vi "Main.vi"() -> ()   [LabVIEW 2023]
panel:
  in  "User interface":T1(tab)
  in  "User entries":enum32{""}(tab)
  in  "Customization":enum32{"Customization"}(tab)
  in  "Marker shape":string
  in  "Marker size":i32
  in  "Open PDF":bool=TRUE
  in  "Open in MATLAB":bool=TRUE
  in  "Colors":enum32{"Colors"}(tab)
  out "Corners":u32(colorbox)
  out "Traces":u32[](array[colorbox])
  in  "Size":enum32{"Size"}(tab)
  out "Depth":i32
  out "Width":i16
  out "Height":i16
  out "stdout":string
  in  "PNG file path":path
  out "PNG picture":picture
  out "Traces.txt":string
  out "Script.m":string
  in  "Arrays":enum32{"Arrays"}(tab)
  out "Pixels colors (uchar)":u32[](array[numeric])
  out "Pixels colors (CLUT)":u8[](array[numeric])
  out "Corners color (CLUT)":i32
  out "Traces colors (RGB)":u8[][](array[numeric])
  out "Traces colors (CLUT)":i32[](array[numeric])
  out "Traces colors string (RGB)":string[](array[string])
  out "Number of Traces":i32
  out "Current VI folder":path
  out "PNG file name":string
  out "Pixmap.bin path":path
  out "Traces.txt path":path
  out "Extract path":path
  out "Script.m path":path
  out "PDF file path":path
  in  "MATLAB":enum32{"CallMATALB"}(tab)
  out "CallMATLAB out":errorcluster
  in  "C 2":enum32{"PNGFile"}(tab)
  out "PNGFile error":errorcluster
  in  "C 3":enum32{"PixmapWrite"}(tab)
  out "PixmapWrite error":errorcluster
  in  "C":enum32{"CallExtract"}(tab)
  out "CallExtract error 2":errorcluster
  out "CallExtract error":errorcluster
  in  "C 4":enum32{"TracesRead"}(tab)
  out "TracesRead error":errorcluster
  in  "C 5":enum32{"ScriptWrite"}(tab)
  out "ScriptWrite error":errorcluster
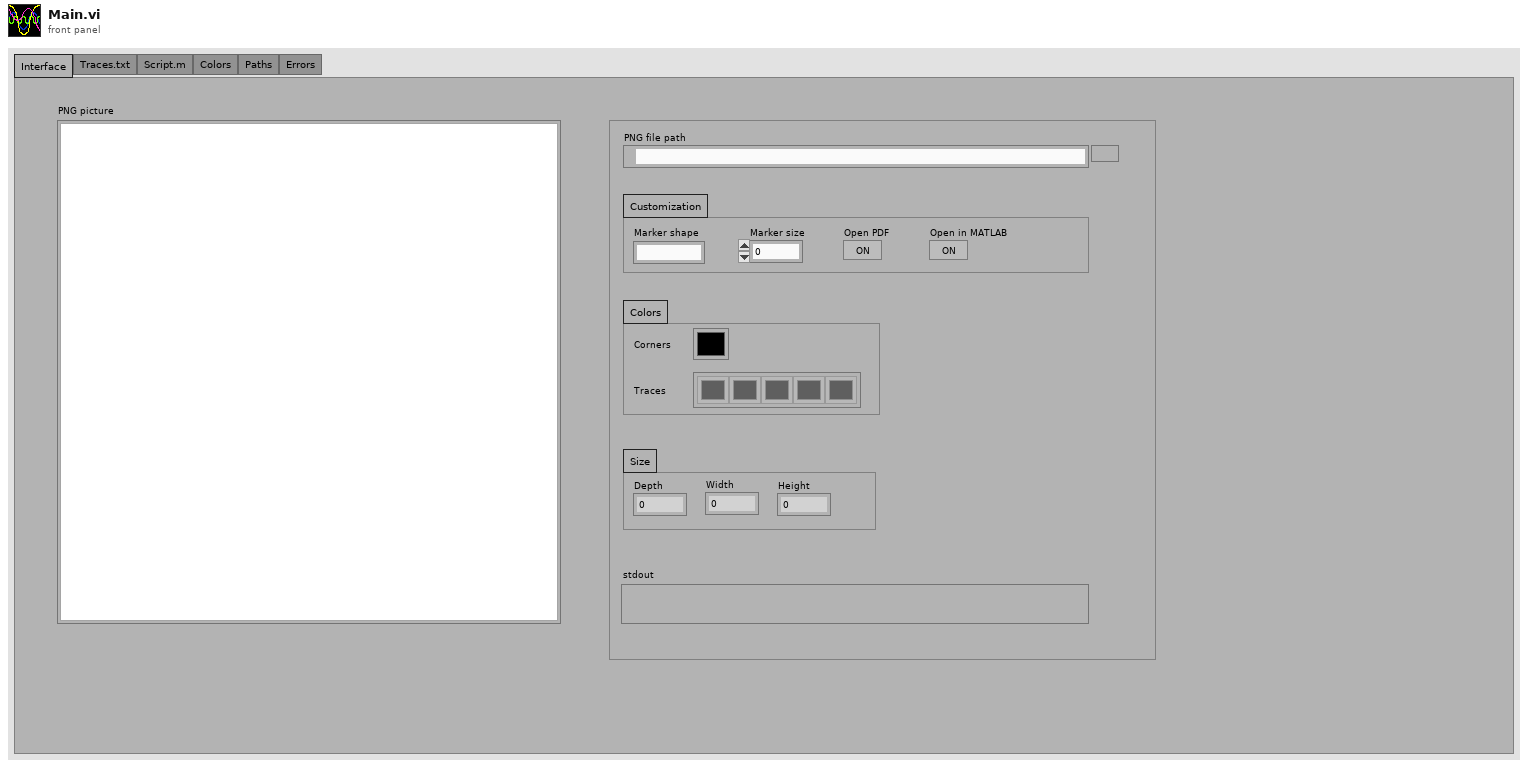
[diagram p1: front panel]
types:
  T1 = enum32{"Interface", "Traces.txt", "Script.m", "Colors", "Paths", "Errors"}
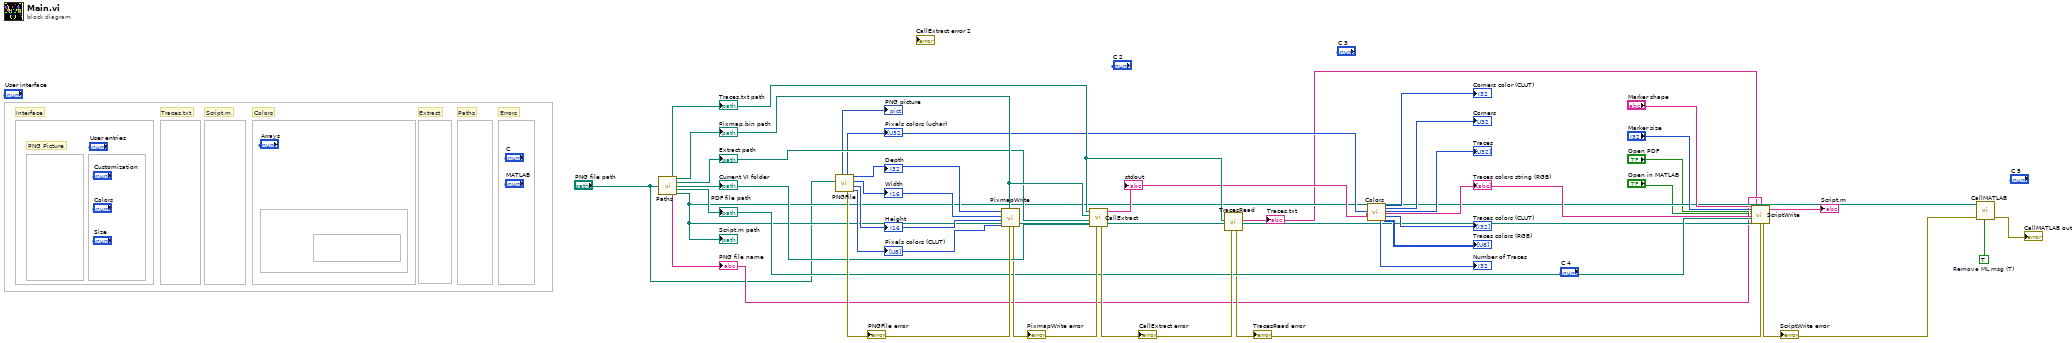
[diagram p0: block diagram]
diagram:
  w34 = TRUE  # Remove ML msg (T)
  # "PNG Picture"
  # "Errors"
  # "Paths"
  # "Extract"
  # "Colors"
  # "Script.m"
  # "Traces.txt"
  # "Interface"
  n1 = call "Paths.vi"("PNG file path"="PNG file path") -> ("Traces.txt path"=w24:path, "Pixmap.bin path"=w28:path, "Extract path"=w27:path, "VI folder"=w26:path, "PDF file path"=w10:path, "PNG file name"=w7:string, "Script.m path"=w9:path)  [unwired: 8 in]
  "Traces.txt path" <- w24
  "Pixmap.bin path" <- w28
  "Extract path" <- w27
  "Current VI folder" <- w26
  "PDF file path" <- w10
  "Script.m path" <- w9
  "PNG file name" <- w7
  n2 = call "PNGFile.vi"("PNG file path"="PNG file path") -> ("Pixels colors (CLUT)"=w30:u8[], "Height"=w31:i16, "Width"=w32:i16, "Depth"=w33:i32, "PNGFile error"=w29:errorcluster, "Pixels colors (uchar)"=w22:u32[], "PNG picture"=→"PNG picture":picture)  [unwired: 4 in]
  "Pixels colors (uchar)" <- w22
  "Depth" <- w33
  "Width" <- w32
  "Height" <- w31
  "Pixels colors (CLUT)" <- w30
  "PNGFile error" <- w29
  n3 = call "PixmapWrite.vi"("PNGFile error in"=w29, "Pixmap.bin path"=w28, "Pixels colors (CLUT)"=w30, "Height"=w31, "Width"=w32, "Depth"=w33) -> ("Pixmap.bin error out"=w25:errorcluster)  [unwired: 5 in]
  "PixmapWrite error" <- w25
  n4 = call "CallExtract.vi"("TracesWrite error"=w25, "VI folder"=w26, "Extract path"=w27, "Pixmap.bin path"=w28, "Traces.txt path"=w24) -> ("stdout"=w21:string, "CallExtract error"=w23:errorcluster)  [unwired: 4 in, 1 out]
  "CallExtract error" <- w23
  "stdout" <- w21
  n5 = call "TracesRead.vi"("Extract error"=w23, "Traces.txt path"=w24) -> ("Traces.txt"=w6:string, "TracesRead error"=w8:errorcluster)  [unwired: 8 in]
  "TracesRead error" <- w8
  "Traces.txt" <- w6
  n6 = call "Colors.vi"("Pixels colors (uchar)"=w22, "stdout"=w21) -> ("Number of Traces"=→"Number of Traces":i32, "Corners color (CLUT)"=→"Corners color (CLUT)":i32, "Corners"=→"Corners":u32, "Traces"=→"Traces":u32[], "Traces colors string (RGB)"=w11:string[], "Traces colors (CLUT)"=→"Traces colors (CLUT)":i32[], "Traces colors (RGB)"=→"Traces colors (RGB)":u8[][])  [unwired: 11 in]
  "Traces colors string (RGB)" <- w11
  n7 = call "ScriptWrite.vi"("Marker shape"="Marker shape", "Marker size"="Marker size", "Open PDF"="Open PDF", "Open in MATLAB"="Open in MATLAB", "Traces colors string (RGB)"=w11, "PDF file path"=w10, "Script.m path"=w9, "Traces.txt"=w6, "TracesRead error"=w8, "PNG file name"=w7) -> ("ScriptWrite error out"=w5:errorcluster, "Script.m"=→"Script.m":string)  [unwired: 16 in]
  "ScriptWrite error" <- w5
  n8 = call "CallMATLAB.vi"("Remove ML msg (T)"=w34, "error in (no error)"=w5, "matlab script path"=w9) -> ("error out"=→"CallMATLAB out":errorcluster)  [unwired: 3 in, 5 out]
